vi "Add Node (recursive).vi"(7 "Section":string[](array[string]), 8 "error in":errorcluster, 9 "Value":variant, 10 "Key":string, 11 "Node in":variant) -> (0 "error out":errorcluster, 3 "Node out":variant)   [LabVIEW 2022 SP3, in "hse-config.lvlib" / "config-base.lvclass"]
doc: "Recursively adds a value node to a section. If section(s) don't exist, it creates them.\n\n____\nHAMPEL SOFTWARE ENGINEERING v3.8.0 (2023-12-18 14:41)"
uses:
  config-base.lvclass
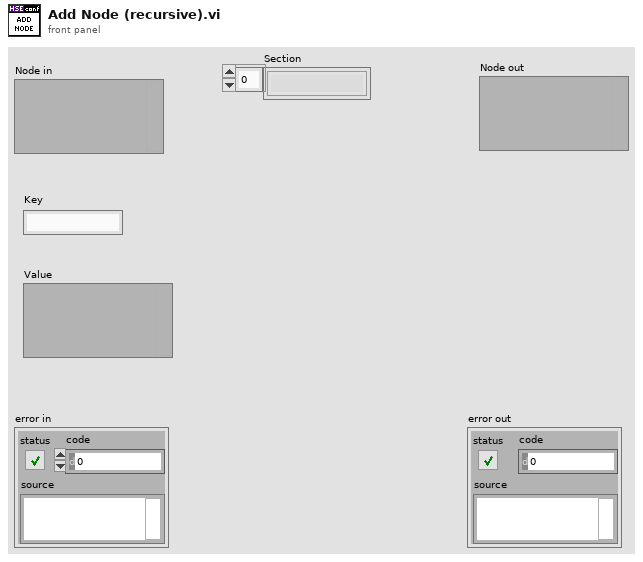
[diagram p1: front panel]
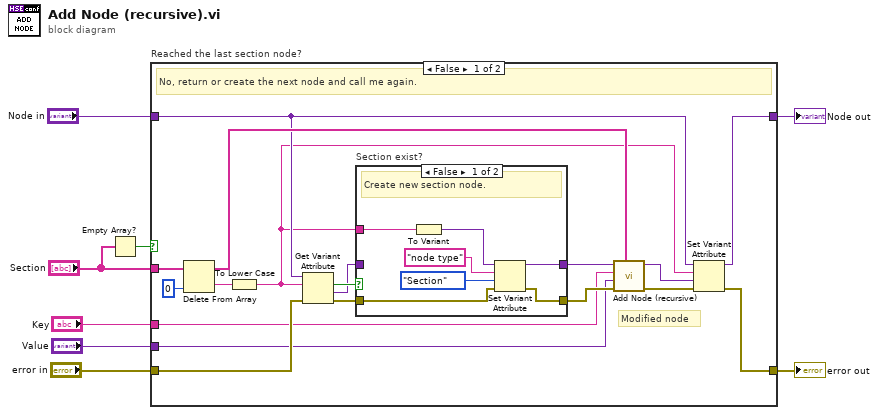
[diagram p0: block diagram]
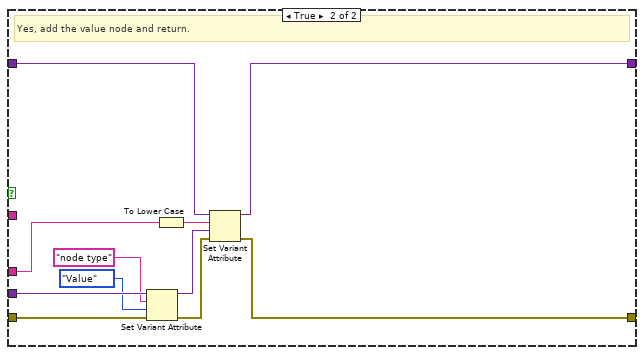
[diagram p3: hidden frame]
diagram:
  n1 = Empty Array?(array="Section") -> (empty?=w6:bool)
  n2 = case "Reached the last section node?" shown="False" w6 {
    tunnel: "error in" -> [w26 w43]
    tunnel: "Node in" -> [w14 w42]
    tunnel: "Value" -> [w21 w46]
    tunnel: "Section" -> [w18 _]
    tunnel: "Key" -> [w16 w39]
    tunnel: [w13 w38] -> w2
    tunnel: [w10 w37] -> w1
    frame False {
      # "Modified node"
      # "No, return or create the next node and call me again."
      n3 = Delete From Array(array=w18, index=0) -> (deleted portion=w11:string, array with subset deleted=w17:string[])  [unwired: 1 in]
      n4 = To Lower Case(string=w11) -> (all lower case string=w9:string)
      n5 = Get Variant Attribute(Variant=w14, name=w9, error in=w26) -> (found=w24:bool, value=w22:variant, error out=w23:errorcluster)  [unwired: 1 in, 1 out]
      n6 = case "Section exist?" shown="False" w24 {
        tunnel: w23 -> [w33 w34]
        tunnel: w22 -> [_ w35]
        tunnel: [w28 w35] -> w20
        tunnel: [w29 w34] -> w25
        tunnel: w9 -> [w27 _]
        frame False {
          # "Create new section node."
          n7 = To Variant(anything=w27) -> (Variant=w31:variant)
          n8 = Set Variant Attribute(Variant=w31, name="node type", value=enum8{"Root", "Section", "Value"}."Section" ("Node Type"), error in=w33) -> (Variant out=w28:variant, error out=w29:errorcluster)  [unwired: 1 out]
        }
        frame True {
          # "Return node."
        }
      }
      n9 = call "Add Node (recursive).vi"("Section"=w17, "error in"=w25, "Value"=w21, "Key"=w16, "Node in"=w20) -> ("error out"=w15:errorcluster, "Node out"=w12:variant)  [unwired: 5 in]
      n10 = Set Variant Attribute(Variant=w14, name=w9, value=w12, error in=w15) -> (Variant out=w13:variant, error out=w10:errorcluster)  [unwired: 1 out]
    }
    frame True {
      # "Yes, add the value node and return."
      n11 = Set Variant Attribute(Variant=w46, name="node type", value=enum8{"Root", "Section", "Value"}."Value" ("Node Type"), error in=w43) -> (Variant out=w40:variant, error out=w41:errorcluster)  [unwired: 1 out]
      n12 = To Lower Case(string=w39) -> (all lower case string=w36:string)
      n13 = Set Variant Attribute(Variant=w42, name=w36, value=w40, error in=w41) -> (Variant out=w38:variant, error out=w37:errorcluster)  [unwired: 1 out]
    }
  }
  "Node out" <- w2
  "error out" <- w1
